vi "Create.vi"(8 "error in (no error)":errorcluster, 10 "gRPC server call":T1, 11 "pin map context":T2) -> (0 "error out":errorcluster, 3 "MeasurementContext out":refnum<class "MeasurementContext.lvclass">)   [LabVIEW 2020, in "CancellableMeasurement.lvlib" / "MeasurementContext.lvclass"]
uses:
  MeasurementContext.lvclass
  RPC Messages/ni_measurementlink_PinMapContext.ctl
  <vilib>/gRPC/LabVIEW gRPC Library/Shared/grpcId.ctl
  MeasurementContext.lvclass/MeasurementContext.ctl
  CancellableMeasurement.lvlib
  <vilib>/gRPC/LabVIEW gRPC Library/grpc-lvsupport-release.lvlib
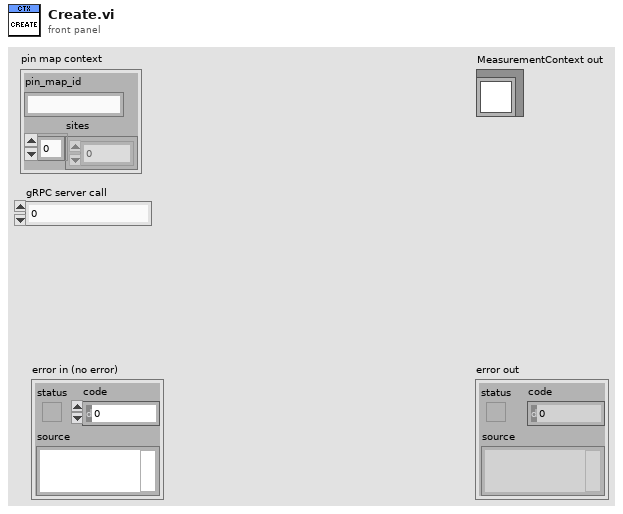
[diagram p1: front panel]
types:
  T1 = typedef "grpc-lvsupport-release.lvlib/grpcId.ctl" = u64
  T2 = typedef "CancellableMeasurement.lvlib/ni_measurementlink_PinMapContext.ctl" = cluster{"pin_map_id":string, "sites":i32[]}
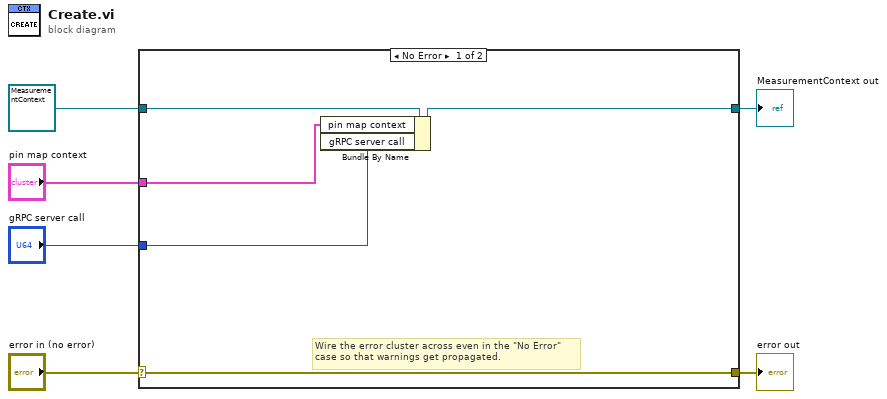
[diagram p0: block diagram]
diagram:
  n1 = case shown="No Error" "error in (no error)" {
    selector: "error in (no error)" -> [w10 w13]
    tunnel: [w10 w13] -> w5
    tunnel: [w9 w12] -> w4
    tunnel: refnum<class "MeasurementContext.lvclass"> refnum ("MeasurementContext.lvclass") -> [w11 w12]
    tunnel: "pin map context" -> [w8 _]
    tunnel: "gRPC server call" -> [w7 _]
    frame No Error {
      # "Wire the error cluster across even in the \"No Error\"\ncase so that warnings get propagated."
      n2 = Bundle By Name(cluster=w11, "pin map context"=w8, "gRPC server call"=w7) -> (w9:refnum<class "MeasurementContext.lvclass">)
    }
    frame Error {
    }
  }
  "error out" <- w5
  "MeasurementContext out" <- w4
